vi "Read ElementType.vi"(8 "error in (no error)":errorcluster, 11 "Tag in":refnum<class "Tag.lvclass">) -> (0 "error out":errorcluster, 2 "ElementType":T1, 3 "Tag out":refnum<class "Tag.lvclass">)   [LabVIEW 2018, in "Tag Engine.lvlib" / "Tag.lvclass"]
uses:
  Tag.lvclass
  <vilib>/Utility/Data Type/Type Definitions/Data Type.ctl
  Tag.lvclass/Tag.ctl
  <vilib>/Utility/Data Type/NI_Data Type.lvlib
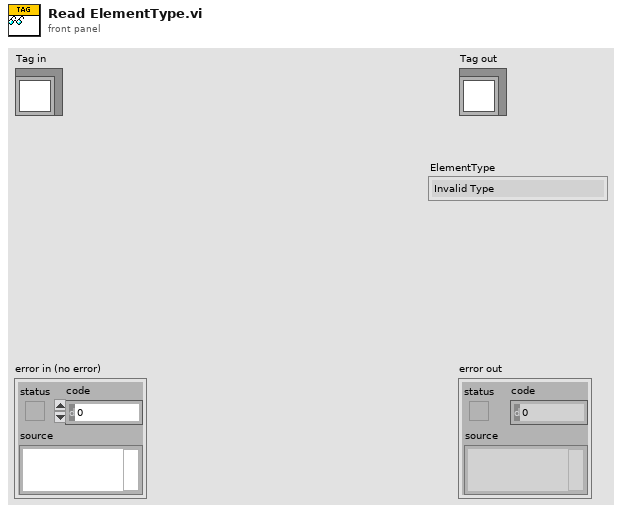
[diagram p1: front panel]
types:
  T1 = typedef "NI_Data Type.lvlib/Data Type.ctl" = enum8{"Invalid Type", "Void", "I8", "I16", "I32", "I64", "U8", "U16", "U32", "U64", "Single Float", "Double Float", "Extended Float", "Single Complex", "Double Complex", "Extended Complex", "Enum U8", "Enum U16", "Enum U32", "Enum U64", "Single Float With Unit", "Double Float With Unit", "Extended Float With Unit", "Single Complex with Unit", "Double Complex with Unit", "Extended Complex with Unit", "Boolean", "String", "Path", "Picture", "Tag", "Array", "Cluster", "Variant", "LV Variant", "Waveform", "Timestamp", "Digital Waveform", "Digital Data", "ExpressData", "Refnum", "External Data", "VI", "Poly VI", "LabVIEW Class Instance", "Fixed Point"}
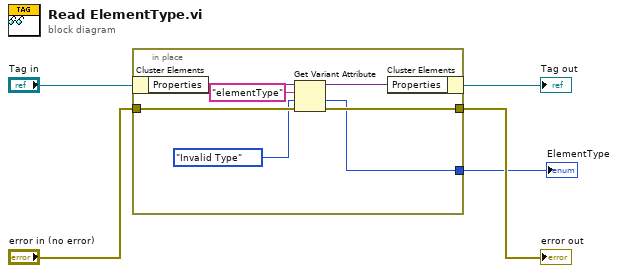
[diagram p0: block diagram]
diagram:
  n1 = in-place {
    in-place-border: "error in (no error)" -> [w9]
    in-place-border: [w8] -> w2
    in-place-border: [w7] -> w1
    n2 = in-place-cluster #1("Tag in") -> ("Properties"=w12:variant)
    n3 = Get Variant Attribute(Variant=w12, name="elementType", default value (empty Variant)=Data_Type."Invalid Type" ("ElementType"), error in=w9) -> (duplicate Variant=w10:variant, value=w7:T1, error out=w8:errorcluster)  [unwired: 1 out]
    n4 = in-place-cluster #1("Properties"=w10) -> (→"Tag out":refnum<class "Tag.lvclass">)
  }
  "error out" <- w2
  "ElementType" <- w1
